vi "Calling Python Script.vi"() -> ()   [LabVIEW 2013]
panel:
  in  "error in":errorcluster
  out "array":dbl[](array[numeric])
  in  "path":path
  in  "Path to Python.exe":path
  out "Raw Python String Output":string
  out "error out":errorcluster
  # "2. Outputs"
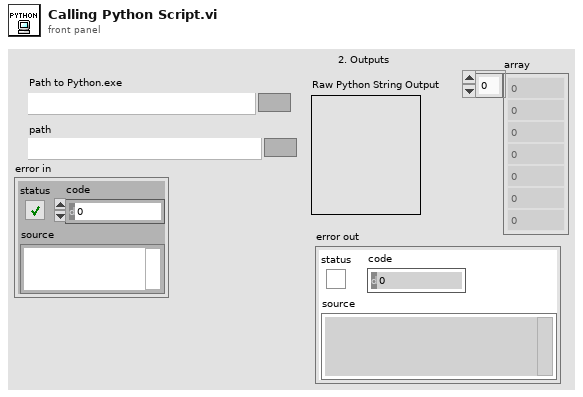
[diagram p1: front panel]
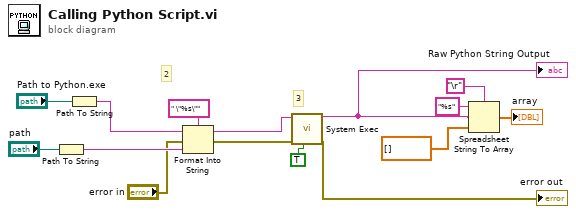
[diagram p0: block diagram]
diagram:
  # "3"
  # "2"
  n1 = Path To String(path="path") -> (string=w14:string)
  n2 = Path To String(path="Path to Python.exe") -> (string=w10:string)
  n3 = Format Into String(format string=" \"%s\"", initial string=w10, error in="error in", w14) -> (resulting string=w13:string, error out=w11:errorcluster)
  n4 = call <vilib>:"System Exec.vi"("run minimized? (F)"=TRUE, "error in (no error)"=w11, "command line"=w13) -> ("error out"=→"error out":errorcluster, "standard output"=w5:string)  [unwired: 5 in, 2 out]
  "Raw Python String Output" <- w5
  n5 = Spreadsheet String To Array(delimiter (Tab)="\r", format string="%s", spreadsheet string=w5, array type (2D Dbl)=dbl[] []) -> (array=→"array":dbl[])
